vi "Encoded String To UTF-8.vi"(8 "error in (no error)":errorcluster, 10 "Encoded string":string, 11 "Encoding in":refnum<class "CConfig UCS-16 Encoding.lvclass">) -> (0 "error out":errorcluster, 2 "UTF-8 string":string, 3 "Encoding out":refnum<class "CConfig UCS-16 Encoding.lvclass">)   [LabVIEW 2013, in "CConfig UCS-16 Encoding.lvclass"]
doc: "Copyright 2018, Carya Automatisering, Wiebe Walstra."
uses:
  CConfig UCS-16 Encoding.lvclass
  CConfig UCS-16 Encoding.lvclass/CConfig UCS-16 Encoding.ctl
  <vilib>/Utility/error.llb/Error Cluster From Error Code.vi
  <vilib>/ErrorRing/Error Ring.xnode
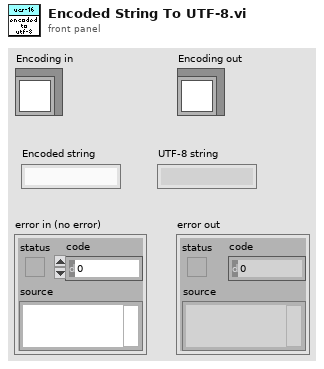
[diagram p1: front panel]
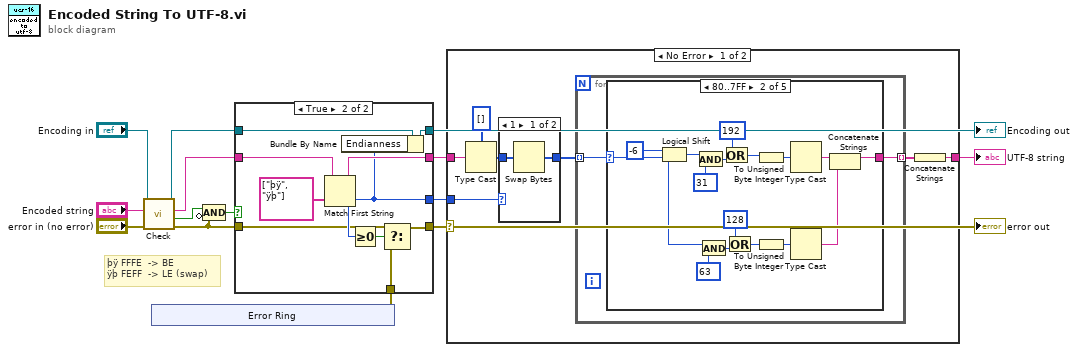
[diagram p0: block diagram]
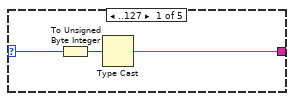
[diagram p3: hidden frame]
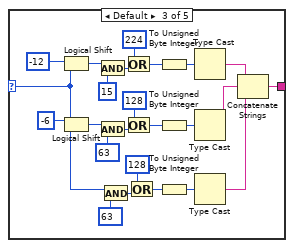
[diagram p4: hidden frame]
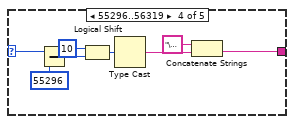
[diagram p5: hidden frame]
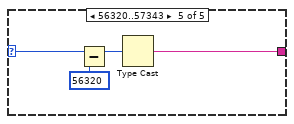
[diagram p6: hidden frame]
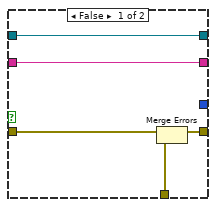
[diagram p8: hidden frame]
diagram:
  # "þÿ FFFE  -> BE\nÿþ FEFF  -> LE (swap)"
  n1 = call-dynamic "Check.vi"("error in (no error)"="error in (no error)", "Encoded string"="Encoded string", "Encoding in"="Encoding in") -> ("error out"=w3:errorcluster, "Match?"=w4:bool, "Encoded string"=w7:string, "Encoding out"=w5:refnum<class "CConfig UCS-16 Encoding.lvclass">)  [unwired: 5 in]
  n2 = xnode "Error Ring"() -> ("error out"=w1:errorcluster)
  n3 = Compound Arithmetic op=AND(w4, invert w3) -> (w2:bool)
  n4 = case shown="True" w2 {
    tunnel: [w16 w29] -> w12
    tunnel: w7 -> [w19 w27]
    tunnel: [w19 w26] -> w11
    tunnel: [w18 w23] -> w14
    tunnel: w5 -> [w18 w24]
    tunnel: [_ w22] -> w10
    tunnel: w3 -> [w17 w21]
    tunnel: w1 -> [w15 w20]
    frame False {
      n5 = Merge Errors(w17, w15) -> (w16:errorcluster)
    }
    frame True {
      n6 = Match First String(2:string[] ["þÿ", "ÿþ"], 3:w27) -> (0:w22:i32, 1:w26:string)
      n7 = Bundle By Name(cluster=w24, "Endianness"=w22) -> (w23:refnum<class "CConfig UCS-16 Encoding.lvclass">)
      n8 = Greater Or Equal To 0?(x=w22) -> (x >= 0?=w25:bool)
      n9 = Select(t=w21, s=w25, f=w20) -> (s? t:f=w29:errorcluster)
    }
  }
  "error out" <- w12
  "Encoding out" <- w14
  n10 = case shown="No Error" w12 {
    tunnel: [w35 w97] -> w13
    tunnel: w11 -> [w31 w97]
    tunnel: w10 -> [w30 _]
    frame No Error {
      n11 = Type Cast(type=u16[] [], x=w31) -> (*(type *) &x=w33:u16[])
      n12 = case shown="1" w30 {
        tunnel: w33 -> [w38 w39]
        tunnel: [w37 w39] -> w32
        frame 1 {
          n13 = Swap Bytes(anything=w38) -> (byte swapped=w37:u16[])
        }
        frame Default {
        }
      }
      n14 = for {
        tunnel: w32 -> [w41] mode=indexing
        tunnel: [w40] -> w36 mode=indexing
        n15 = case shown="80..7FF" w41 {
          selector: w41 -> [w44 w46 w63 w92 w96]
          tunnel: [w42 w60 w84 w85 w93] -> w40
          frame ..127 {
            n16 = To Unsigned Byte Integer(number=w44) -> (unsigned 8bit integer=w43:u8)
            n17 = Type Cast(x=w43) -> (*(type *) &x=w42:string)  [unwired: 1 in]
          }
          frame 128..2047 {
            n18 = Logical Shift(y=i16 -6, x=w46) -> (x << y=w57:u16)
            n19 = And(x=w57, y=u16 31) -> (x .and. y?=w55:u16)
            n20 = And(x=w46, y=u16 63) -> (x .and. y?=w48:u16)
            n21 = Or(x=u16 192 ("y"), y=w55) -> (x .or. y?=w53:u16)
            n22 = Or(x=u16 128 ("y"), y=w48) -> (x .or. y?=w50:u16)
            n23 = To Unsigned Byte Integer(number=w53) -> (unsigned 8bit integer=w52:u8)
            n24 = To Unsigned Byte Integer(number=w50) -> (unsigned 8bit integer=w51:u8)
            n25 = Type Cast(x=w52) -> (*(type *) &x=w59:string)  [unwired: 1 in]
            n26 = Type Cast(x=w51) -> (*(type *) &x=w45:string)  [unwired: 1 in]
            n27 = Concatenate Strings(w59, w45) -> (w60:string)
          }
          frame Default {
            n28 = Logical Shift(y=i16 -12, x=w63) -> (x << y=w82:u16)
            n29 = Logical Shift(y=i16 -6, x=w63) -> (x << y=w65:u16)
            n30 = And(x=w82, y=u16 15) -> (x .and. y?=w80:u16)
            n31 = And(x=w65, y=u16 63) -> (x .and. y?=w67:u16)
            n32 = And(x=w63, y=u16 63) -> (x .and. y?=w73:u16)
            n33 = Or(x=u16 224 ("y"), y=w80) -> (x .or. y?=w78:u16)
            n34 = Or(x=u16 128 ("y"), y=w67) -> (x .or. y?=w69:u16)
            n35 = Or(x=u16 128 ("y"), y=w73) -> (x .or. y?=w75:u16)
            n36 = To Unsigned Byte Integer(number=w78) -> (unsigned 8bit integer=w77:u8)
            n37 = To Unsigned Byte Integer(number=w69) -> (unsigned 8bit integer=w70:u8)
            n38 = To Unsigned Byte Integer(number=w75) -> (unsigned 8bit integer=w76:u8)
            n39 = Type Cast(x=w77) -> (*(type *) &x=w83:string)  [unwired: 1 in]
            n40 = Type Cast(x=w70) -> (*(type *) &x=w62:string)  [unwired: 1 in]
            n41 = Type Cast(x=w76) -> (*(type *) &x=w71:string)  [unwired: 1 in]
            n42 = Concatenate Strings(w83, w62, w71) -> (w84:string)
          }
          frame 55296..56319 {
            n43 = Subtract(x=w92, y=u16 55296) -> (x-y=w90:u16)
            n44 = Logical Shift(y=i16 10, x=w90) -> (x << y=w88:u16)
            n45 = Type Cast(x=w88) -> (*(type *) &x=w87:string)  [unwired: 1 in]
            n46 = Concatenate Strings("\u0001" ("string"), w87) -> (w85:string)
          }
          frame 56320..57343 {
            n47 = Subtract(x=w96, y=u16 56320) -> (x-y=w94:u16)
            n48 = Type Cast(x=w94) -> (*(type *) &x=w93:string)  [unwired: 1 in]
          }
        }
      }
      n49 = Concatenate Strings(w36) -> (w35:string)
    }
    frame Error {
    }
  }
  "UTF-8 string" <- w13
